vi "parseValue.vi"(8 "error in (no error)":errorcluster, 10 "message":string, 11 "AlCS in":refnum<class "AlCS.lvclass">) -> (0 "error out":errorcluster, 1 "value":variant, 2 "data":T1, 3 "AlCS out":refnum<class "AlCS.lvclass">)   [LabVIEW 2016, in "AlCS.lvclass"]
uses:
  AlCS.lvclass
  Typedefs/data.ctl
  ts_monochromator_windows/Typedefs/publishers.ctl
  ts_monochromator_windows/Typedefs/GratingType.ctl
  ts_monochromator_windows/Typedefs/slitWidth.ctl
  ts_monochromator_windows/Typedefs/DeviceStatus.ctl
  ts_monochromator_windows/Typedefs/AckType.ctl
  ts_monochromator_windows/Typedefs/wavelength.ctl
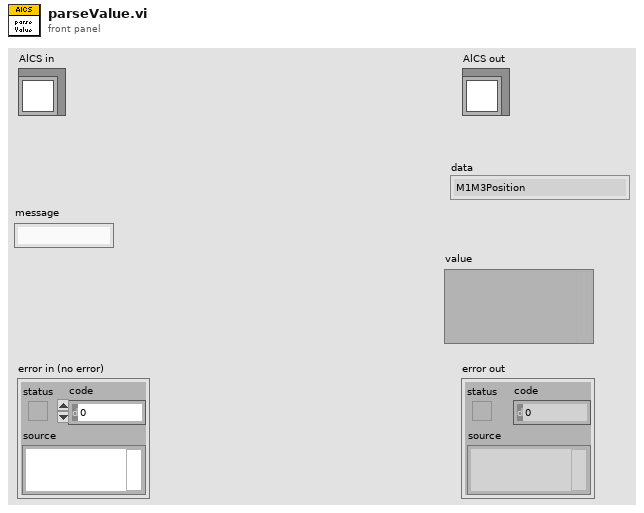
[diagram p1: front panel]
types:
  T1 = typedef "data.ctl" = enum16{"M1M3Position", "M2Position", "CameraPosition", "LaserStatus", "DeviceStatus", "Ack"}
  T2 = typedef "publishers.ctl" = enum16{"Wavelength", "Grating", "FrontEntranceSlitPosition", "FrontExitSlitPosition", "SoftwareStatus", "MonochromatorId", "Ack"}
  T3 = typedef "GratingType.ctl" = enum16{"Blue", "Red", "Mirror"}
  T4 = typedef "slitWidth.ctl" = dbl
  T5 = typedef "DeviceStatus.ctl" = enum16{"SettingUp", "Ready", "Offline", "Fault"}
  T6 = typedef "AckType.ctl" = enum16{"OK", "OutOfRange", "Unknown", "Busy", "Rejected"}
  T7 = typedef "wavelength.ctl" = dbl
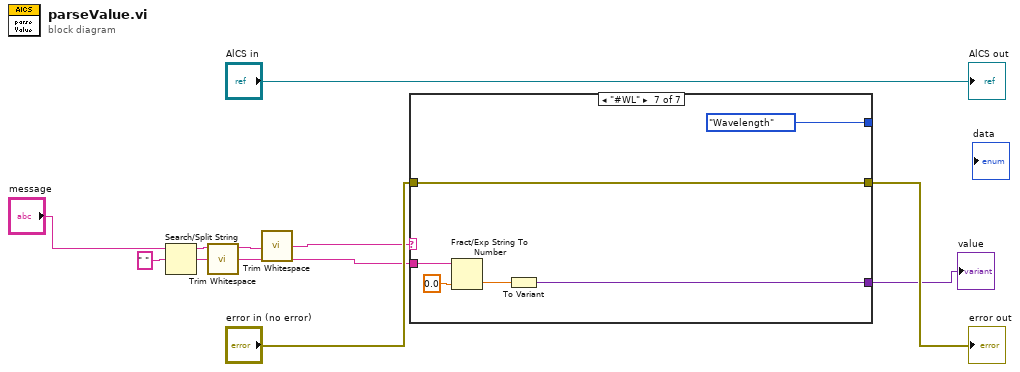
[diagram p0: block diagram]
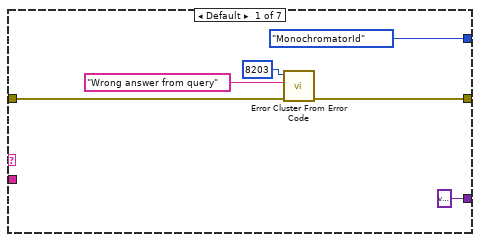
[diagram p2: hidden frame]
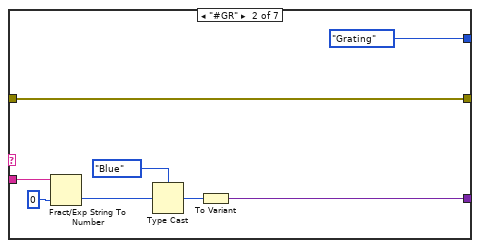
[diagram p3: hidden frame]
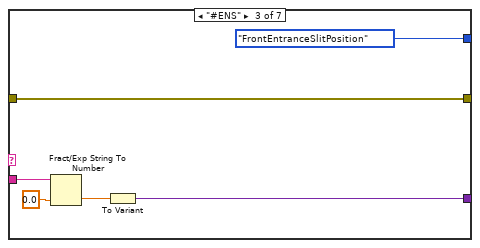
[diagram p4: hidden frame]
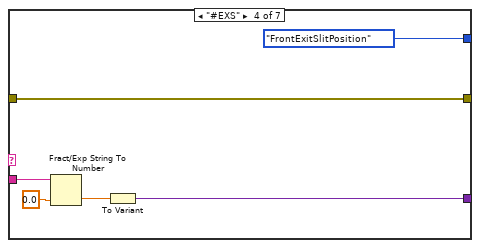
[diagram p5: hidden frame]
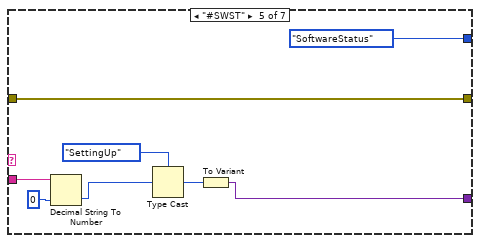
[diagram p6: hidden frame]
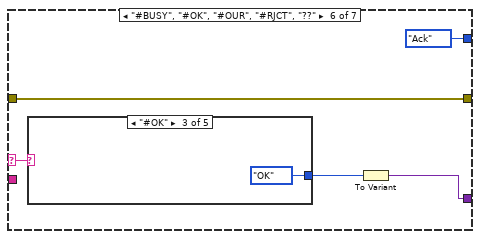
[diagram p7: hidden frame]
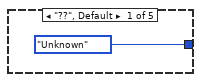
[diagram p8: hidden frame]
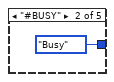
[diagram p9: hidden frame]
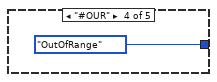
[diagram p10: hidden frame]
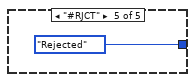
[diagram p11: hidden frame]
diagram:
  n1 = Search/Split String(string="message", search string/char (-)=" ") -> (substring before match=w7:string, match + rest of string=w6:string)  [unwired: 1 in, 1 out]
  n2 = call <vilib>:"Trim Whitespace.vi"("string"=w6) -> ("trimmed string"=w2:string)  [unwired: 1 in]
  n3 = call <vilib>:"Trim Whitespace.vi"("string"=w7) -> ("trimmed string"=w3:string)  [unwired: 1 in]
  n4 = case shown="\"#WL\"" w3 {
    selector: w3 -> [_ _ _ _ _ w46 _]
    tunnel: w2 -> [_ w23 w27 w33 w44 _ w60]
    tunnel: [variant ("Variant") w24 w29 w35 w40 w47 w57] -> w1
    tunnel: "error in (no error)" -> [w15 w17 w25 w31 w38 w49 w55]
    tunnel: [w14 w17 w25 w31 w38 w49 w55] -> w8
    tunnel: [publishers."MonochromatorId" ("publishers") publishers."Grating" ("publishers") publishers."FrontEntranceSlitPosition" ("publishers") publishers."FrontExitSlitPosition" ("publishers") publishers."SoftwareStatus" ("publishers") publishers."Ack" ("publishers") publishers."Wavelength" ("publishers")] -> _
    frame Default {
      n5 = call <vilib>:"Error Cluster From Error Code.vi"("error in (no error)"=w15, "error message (\"\")"="Wrong answer from query" ("error message (\"\")"), "error code (0)"=8203) -> ("error out"=w14:errorcluster)  [unwired: 6 in]
    }
    frame "#GR" {
      n6 = Fract/Exp String To Number(string=w23, default (0 dbl)=u16 0) -> (number=w20:u16)  [unwired: 2 in, 1 out]
      n7 = Type Cast(type=GratingType."Blue" ("GratingType"), x=w20) -> (*(type *) &x=w21:T3)
      n8 = To Variant(anything=w21) -> (Variant=w24:variant)
    }
    frame "#ENS" {
      n9 = Fract/Exp String To Number(string=w27, default (0 dbl)=T4 0.0 ("position")) -> (number=w30:dbl)  [unwired: 2 in, 1 out]
      n10 = To Variant(anything=w30) -> (Variant=w29:variant)
    }
    frame "#EXS" {
      n11 = Fract/Exp String To Number(string=w33, default (0 dbl)=T4 0.0 ("position")) -> (number=w36:dbl)  [unwired: 2 in, 1 out]
      n12 = To Variant(anything=w36) -> (Variant=w35:variant)
    }
    frame "#SWST" {
      n13 = Decimal String To Number(string=w44, default (0L)=u16 0 ("default (0 I32)")) -> (number=w37:u16)  [unwired: 1 in, 1 out]
      n14 = Type Cast(type=DeviceStatus."SettingUp" ("DeviceStatus"), x=w37) -> (*(type *) &x=w41:T5)
      n15 = To Variant(anything=w41) -> (Variant=w40:variant)
    }
    frame "#BUSY", "#OK", "#OUR", "#RJCT", "??" {
      n16 = case shown="\"#OK\"" w46 {
        tunnel: [AckType."Unknown" ("Ack") AckType."Busy" ("Ack") AckType."OK" ("Ack") AckType."OutOfRange" ("Ack") AckType."Rejected" ("Ack")] -> w45
        frame "??", Default {
        }
        frame "#BUSY" {
        }
        frame "#OK" {
        }
        frame "#OUR" {
        }
        frame "#RJCT" {
        }
      }
      n17 = To Variant(anything=w45) -> (Variant=w47:variant)
    }
    frame "#WL" {
      n18 = Fract/Exp String To Number(string=w60, default (0 dbl)=T7 0.0 ("wavelength")) -> (number=w58:dbl)  [unwired: 2 in, 1 out]
      n19 = To Variant(anything=w58) -> (Variant=w57:variant)
    }
  }
  "error out" <- w8
  "value" <- w1
  "AlCS out" <- "AlCS in"
